vi "placeBottom.vi"(4 "spacing[pixel]":u16, 6 "useControlBodyOnly":bool, 8 "error in (no error)":errorcluster, 10 "anchorObject":refnum<vi>, 11 "movingObject":refnum<vi>) -> (0 "error out":errorcluster, 2 "anchorObject(dup)":refnum<vi>, 3 "movingObject(dup)":refnum<vi>)   [LabVIEW 2023]
doc: "Places the 'movingObject' under the 'anchorObject' with the given spacing.\n\nThe operation affects only the Y coordinate.\nThe X coordinate of the item is not modified."
uses:
  Misc/hideCaption&Label.vi
  Misc/setCaption&LabelVisibility.vi
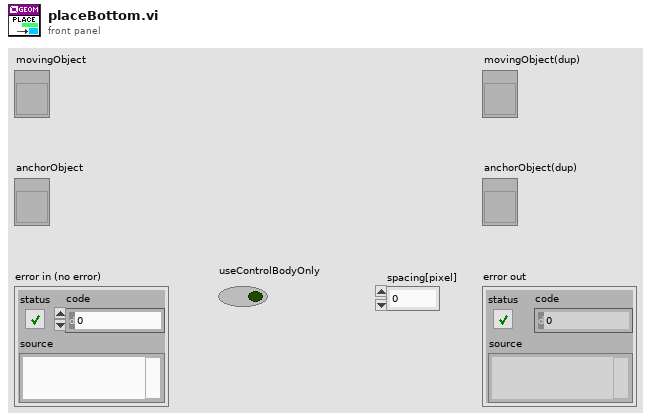
[diagram p1: front panel]
types:
  T1 = cluster{"left":i32, "top":i32, "right":i32, "bottom":i32}
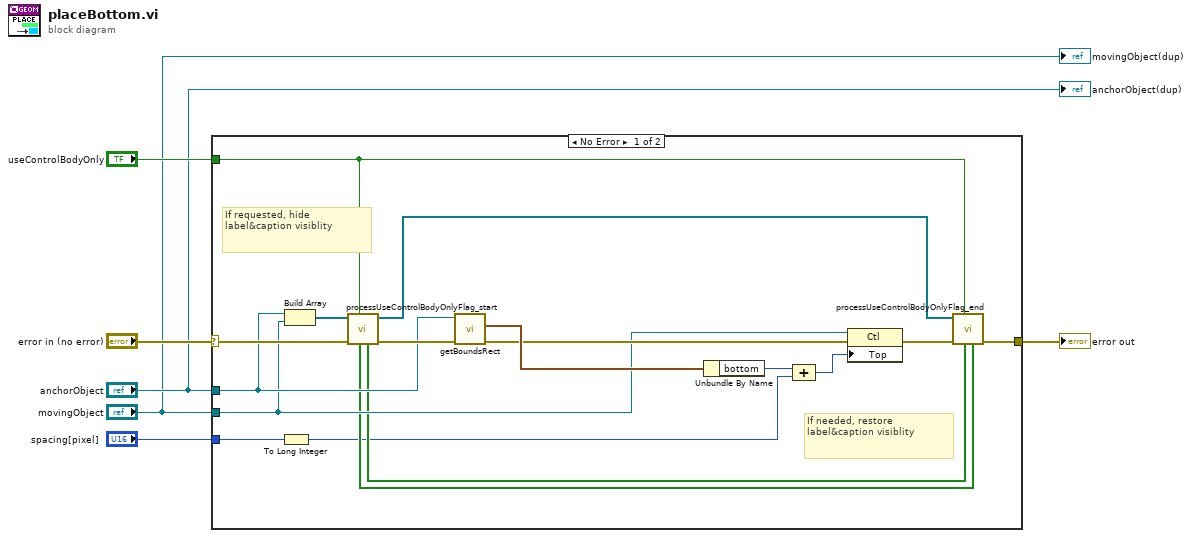
[diagram p0: block diagram]
diagram:
  n1 = case shown="No Error" "error in (no error)" {
    selector: "error in (no error)" -> [w23 w24]
    tunnel: [w20 w24] -> w6
    tunnel: "anchorObject" -> [w18 _]
    tunnel: "useControlBodyOnly" -> [w10 _]
    tunnel: "movingObject" -> [w15 _]
    tunnel: "spacing[pixel]" -> [w13 _]
    frame No Error {
      # "If needed, restore label&caption visiblity"
      # "If requested, hide label&caption visiblity"
      n2 = To Long Integer(number=w13) -> (32bit integer=w7:i32)
      n3 = Build Array(w18, w15) -> (w22:refnum<vi>[])
      n4 = call "processUseControlBodyOnlyFlag_start.vi"("useControlBodyOnly"=w10, "error in (no error)"=w23, "refList"=w22) -> ("error out"=w19:errorcluster, "refList(dup)"=w21:refnum<vi>[], "LabelVisibilityList"=w9:bool[], "captionVisibilityList"=w8:bool[])  [unwired: 5 in]
      n5 = call "getBoundsRect.vi"("error in (no error)"=w19, "ref"=w18) -> ("error out"=w16:errorcluster, "rect"=w17:T1)  [unwired: 7 in, 1 out]
      n6 = Unbundle By Name(w17) -> ("bottom"=w14:i32)
      n7 = Compound Arithmetic op=ADD(w14, w7) -> (w11:i32)
      n8 = property class="Ctl"(reference=w15, error in=w16, "Top"=w11) -> (error out=w12:errorcluster)  [unwired: 1 out]
      n9 = call "processUseControlBodyOnlyFlag_end.vi"("captionVisibilityList"=w8, "LabelVisibilityList"=w9, "useControlBodyOnly"=w10, "error in (no error)"=w12, "refList"=w21) -> ("error out"=w20:errorcluster)  [unwired: 5 in, 1 out]
    }
    frame Error {
    }
  }
  "error out" <- w6
  "movingObject(dup)" <- "movingObject"
  "anchorObject(dup)" <- "anchorObject"
